vi "Write Send Headers.vi"(8 "error in (no error)":errorcluster, 10 "additional send headers (none)":T1[](array[typedef]), 11 "WebSockets in":refnum<class "WebSocket.lvclass">) -> (0 "error out":errorcluster, 3 "WebSockets out":refnum<class "WebSocket.lvclass">)   [LabVIEW 2013, in "WebSockets.lvlib" / "WebSocket.lvclass"]
uses:
  WebSocket.lvclass
  Headers.ctl
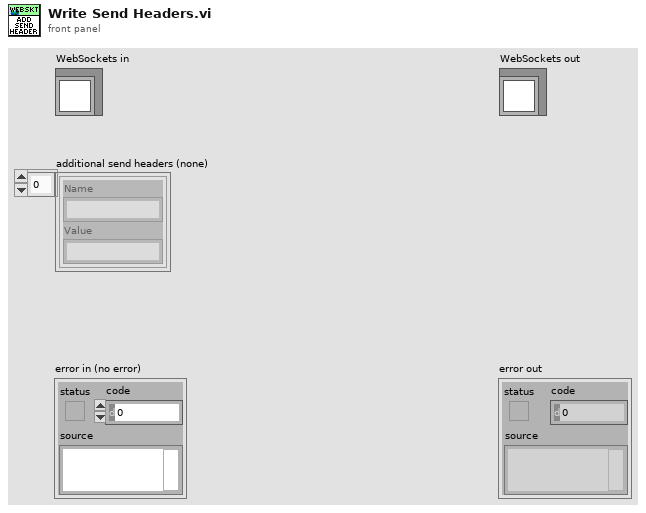
[diagram p1: front panel]
types:
  T1 = typedef "WebSockets.lvlib/WebSocket.lvclass/Headers.ctl" = cluster{"Name":string, "Value":string}
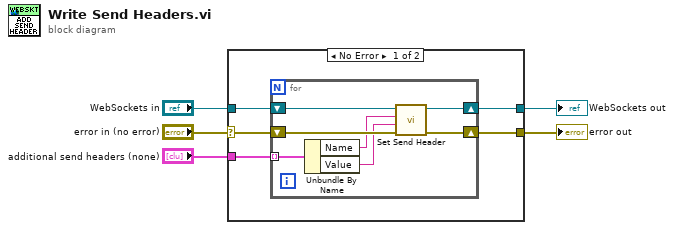
[diagram p0: block diagram]
diagram:
  n1 = case shown="No Error" "error in (no error)" {
    selector: "error in (no error)" -> [w7 w19]
    tunnel: [w6 w19] -> w4
    tunnel: [w8 w18] -> w2
    tunnel: "WebSockets in" -> [w9 w18]
    tunnel: "additional send headers (none)" -> [w10 _]
    frame No Error {
      n2 = for {
        tunnel: w10 -> [w13] mode=indexing
        shift-right: [w16] -> w8
        shift-left: w9 -> [w17]
        shift-right: [w14] -> w6
        shift-left: w7 -> [w15]
        n3 = Unbundle By Name(w13) -> ("Name"=w12:string, "Value"=w11:string)
        n4 = call "Set Send Header.vi"("error in (no error)"=w15, "Value"=w11, "Name"=w12, "WebSockets in"=w17) -> ("error out"=w14:errorcluster, "WebSockets out"=w16:refnum<class "WebSocket.lvclass">)  [unwired: 6 in]
      }
    }
    frame Error {
    }
  }
  "error out" <- w4
  "WebSockets out" <- w2
